vi "Find Start and Endpoint Body Text.vi"(11 "Icon":picture) -> (1 "Pos offset":i32, 2 "Neg offset":i32, 3 "Found?":bool, 5 "Transparent?":bool)   [LabVIEW 2021, in "lv_icon.lvlib"]
doc: "Find the actual start and endpoint of the text to be able to center the Text later on."
uses:
  lv_icon.lvlib
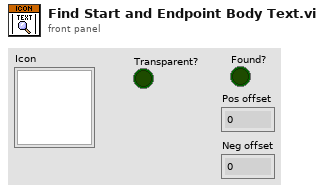
[diagram p1: front panel]
types:
  T1 = cluster{"left":i16, "top":i16, "right":i16, "bottom":i16}
  T2 = typedef "imagedata.ctl" = cluster{"image type":i32, "image depth":i32, "image":u8[], "mask":u8[], "colors":u32[], "Rectangle":cluster{"left":i16, "top":i16, "right":i16, "bottom":i16}}
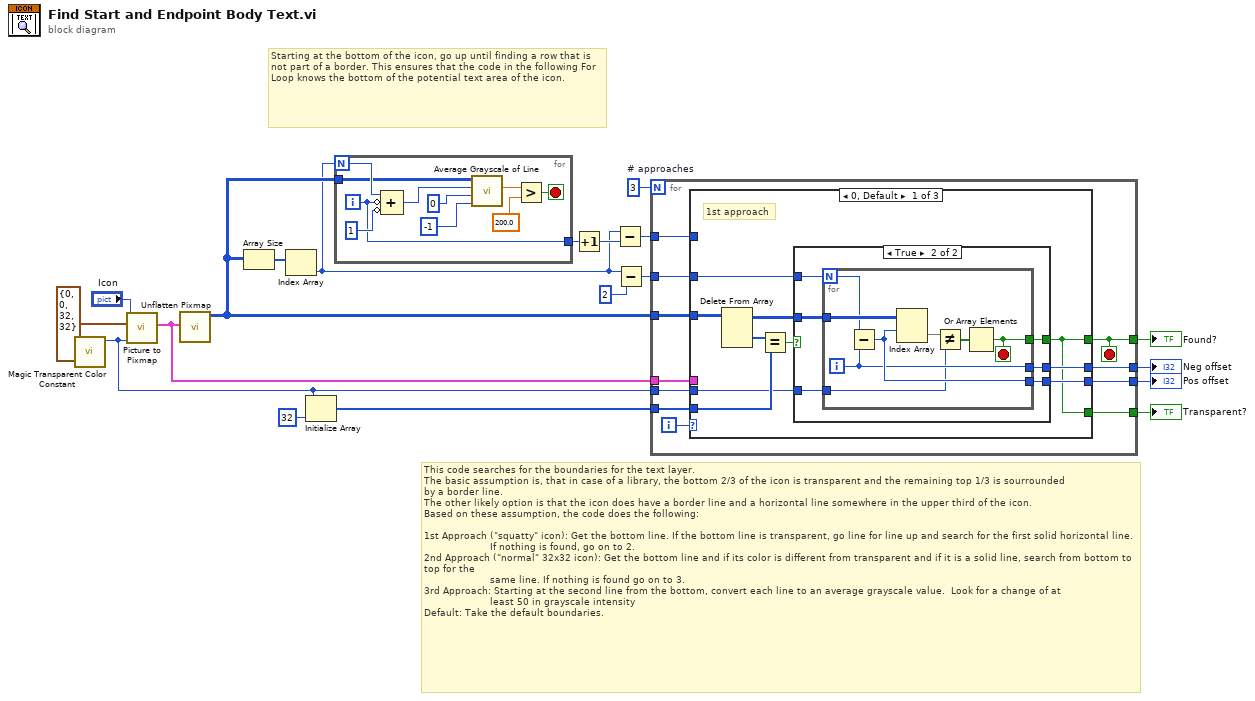
[diagram p0: block diagram]
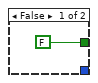
[diagram p2: hidden frame]
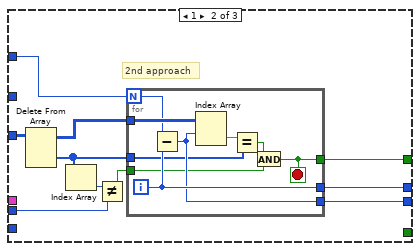
[diagram p3: hidden frame]
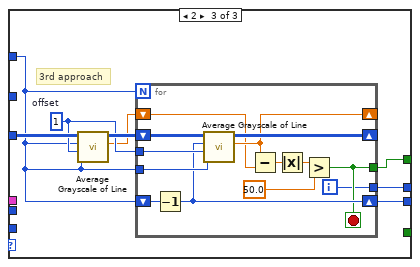
[diagram p4: hidden frame]
diagram:
  w17 = 3  # # approaches
  # "Starting at the bottom of the icon, go up until finding a row that is not part of a border. This ensures that the code in the following For Loop knows the bottom of the potential text area of the icon."
  # "This code searches for the boundaries for the text layer.\nThe basic assumption is, that in case of a library, the bottom 2/3 of the icon is transparent and the remaining top 1/3 is sourrounded\nby a border line.\nThe other likely option is that the icon does have a border line and a horizontal line somewhere in the upper third of the icon.\nBased on these assumption, the code does the following:\n\n1st Approach (\"squatty\" icon): Get the bottom line. If the bottom line is transparent, go line for line up and search for the first solid horizontal line.\n                      If nothing is found, go on to 2.\n2nd Approach (\"normal\" 32x32 icon): Get the bottom line and if its color is different from transparent and if it is a solid line, search from bottom to top for the\n                      same line. If nothing is found go on to 3. \n3rd Approach: Starting at the second line from the bottom, convert each line to an average grayscale value.  Look for a change of at\n                      least 50 in grayscale intensity\nDefault: Take the default boundaries."
  n1 = call "Magic Transparent Color Constant.vi"() -> ("Magic transparent color constant"=w7:u32)  [unwired: 11 out]
  n2 = call <vilib>:"Picture to Pixmap.vi"("Background Color"=w7, "rect"=T1 {"left"=0, "top"=0, "right"=32, "bottom"=32}, "picture"="Icon") -> ("image data"=w11:T2)  [unwired: 1 in, 7 out]
  n3 = call <vilib>:"Unflatten Pixmap.vi"("image data"=w11) -> ("24-bit pixmap"=w4:u32[][])  [unwired: 10 out]
  n4 = Array Size(array=w4) -> (size(s)=w16:i32[])
  n5 = Index Array(array=w16) -> (element=w2:i32)  [unwired: 1 in]
  n6 = Initialize Array(w7, 32 ("dimension size")) -> (w8:u32[])
  n7 = for {
    N: w2 -> [w29]
    tunnel: w4 -> [w26]
    tunnel: [w27] -> w5
    i -> [w27]
    stop <- w22 stop-if-true
    n8 = Compound Arithmetic op=ADD(w29, invert w27, invert 1) -> (w25:i32)
    n9 = call "Average Grayscale of Line.vi"("nPoints"=-1, "offset"=0, "row"=w25, "24-bit pixmap in"=w26) -> ("average grayscale"=w24:sgl)  [unwired: 6 in, 1 out]
    n10 = Greater?(x=w24, y=sgl 200.0) -> (0:w22:bool)
  }
  n11 = Increment(x=w5) -> (x+1=w3:i32)
  n12 = Subtract(x=w2, y=w3) -> (x-y=w1:i32)
  n13 = Subtract(x=w2, y=2) -> (x-y=w14:i32)
  n14 = for {
    N: w17 -> [_]
    tunnel: [w40] -> w12
    tunnel: [w36] -> w19
    tunnel: w14 -> [w39]
    tunnel: [w38] -> w13
    tunnel: w4 -> [w37]
    tunnel: w11 -> [w35]
    tunnel: w8 -> [w33]
    tunnel: w7 -> [w32]
    tunnel: [w31] -> w6
    tunnel: w1 -> [w30]
    i -> [w34]
    stop <- w36 stop-if-true
    n15 = case shown="0, Default" w34 {
      tunnel: [w48 w75 w92] -> w40
      tunnel: [w42 w74 w87] -> w36
      tunnel: w39 -> [w41 _ _]
      tunnel: [w49 w73 w86] -> w38
      tunnel: w37 -> [w50 w71 w90]
      tunnel: w35 -> [_ _ _]
      tunnel: w33 -> [w47 _ _]
      tunnel: w32 -> [w46 w68 _]
      tunnel: [w42 _ _] -> w31
      tunnel: w30 -> [_ w66 w85]
      frame 0, Default {
        # "1st approach"
        n16 = Delete From Array(array=w50) -> (deleted portion=w45:u32[], array with subset deleted=w43:u32[][])  [unwired: 3 in]
        n17 = Equal?(x=w45, y=w47) -> (x = y?=w44:bool)
        n18 = case shown="True" w44 {
          tunnel: w43 -> [_ w56]
          tunnel: w41 -> [_ w57]
          tunnel: [FALSE w55] -> w42
          tunnel: [_ w54] -> w49
          tunnel: [_ w53] -> w48
          tunnel: w46 -> [_ w52]
          frame False {
          }
          frame True {
            n19 = for {
              N: w57 -> [w63]
              tunnel: w56 -> [w65]
              tunnel: [w60] -> w55
              tunnel: [w62] -> w54
              tunnel: [w64] -> w53
              tunnel: w52 -> [w58]
              i -> [w62]
              stop <- w60 stop-if-true
              n20 = Subtract(x=w63, y=w62) -> (x-y=w64:i32)
              n21 = Index Array(array=w65, index (row)=w64) -> (element=w61:u32[])  [unwired: 1 in]
              n22 = Not Equal?(x=w61, y=w58) -> (x != y?=w59:bool[])
              n23 = Or Array Elements(Boolean array=w59) -> (logical OR=w60:bool)
            }
          }
        }
      }
      frame 1 {
        # "2nd approach"
        n24 = Delete From Array(array=w71) -> (deleted portion=w69:u32[], array with subset deleted=w72:u32[][])  [unwired: 3 in]
        n25 = Index Array(array=w69) -> (element=w70:u32)  [unwired: 1 in]
        n26 = Not Equal?(x=w70, y=w68) -> (x != y?=w67:bool)
        n27 = for {
          N: w66 -> [w80]
          tunnel: w72 -> [w84]
          tunnel: w69 -> [w77]
          tunnel: [w78] -> w74
          tunnel: [w83] -> w73
          tunnel: [w81] -> w75
          tunnel: w67 -> [w76]
          i -> [w83]
          stop <- w78 stop-if-true
          n28 = Subtract(x=w80, y=w83) -> (x-y=w81:i32)
          n29 = Index Array(array=w84, index (row)=w81) -> (element=w82:u32[])  [unwired: 1 in]
          n30 = Equal?(x=w82, y=w77) -> (x = y?=w79:bool)
          n31 = And(x=w79, y=w76) -> (x .and. y?=w78:bool)
        }
      }
      frame 2 {
        w89 = 1  # offset
        # "3rd approach"
        n32 = call "Average Grayscale of Line.vi"("nPoints"=w85, "offset"=w89, "row"=w85, "24-bit pixmap in"=w90) -> ("average grayscale"=w88:sgl, "24-bit pixmap out"=w91:u32[][])  [unwired: 6 in]
        n33 = for {
          N: w85 -> [_]
          shift-right: [w100] -> _
          shift-left: w91 -> [w105]
          shift-right: [w101] -> w92
          shift-left: w85 -> [w104]
          tunnel: w85 -> [w102]
          tunnel: w89 -> [w103]
          shift-right: [w99] -> _
          shift-left: w88 -> [w98]
          tunnel: [w94] -> w87
          tunnel: [w93] -> w86
          i -> [w93]
          stop <- w94 stop-if-true
          n34 = Decrement(x=w104) -> (x-1=w101:i32)
          n35 = call "Average Grayscale of Line.vi"("nPoints"=w102, "offset"=w103, "row"=w101, "24-bit pixmap in"=w105) -> ("average grayscale"=w99:sgl, "24-bit pixmap out"=w100:u32[][])  [unwired: 6 in]
          n36 = Subtract(x=w99, y=w98) -> (x-y=w97:sgl)
          n37 = Absolute Value(x=w97) -> (abs(x)=w96:sgl)
          n38 = Greater?(x=w96, y=sgl 50.0) -> (0:w94:bool)
        }
      }
    }
  }
  "Pos offset" <- w12
  "Found?" <- w19
  "Neg offset" <- w13
  "Transparent?" <- w6
